vi "Playing with Octave Bands.vi"() -> ()   [LabVIEW 2014]
uses:
  <vilib>/Analysis/baseanly.llb/Mean (DBL).vi
  <vilib>/measure/maspectr.llb/FFT Spectrum (Mag-Phase) for 1 Chan.vi
  <vilib>/Analysis/NI_AALBase.lvlib
  <vilib>/Analysis/NI_AALPro.lvlib
  <vilib>/measure/NI_MAPro.lvlib
panel:
  in  "bandwidth":T1(ring)=enum."1/3 octave"
  in  "Octave":dbl=0.33 format="%#_13g"
  out "Mic Spectrum 3":cluster{"Fctr":ext[], "magnitude":dbl[]}[](graph)=[{"Fctr"=[25.73721928961165, 32.352028870043036, 40.66693298256041, 51.11887865986131, 64.25711416600414, 80.77205191484325, 101.53154954452943, 127.62651571339914, 160.428237195363, 201.66043980553155, 253.48986994750726, 318.6401568298155, 400.534938794811, 503.47777502835936, 632.87829698514, 795.5364837549187, 1000.0, 1257.0133745218284, 1580.0826237267545, 1986.1849908740721, 2496.6610978032245, 3138.3363915870036, 3944.9308179734376, 4958.830799755948, 6233.3166372840005, 7835.362380695417, 9849.155306759334, 12380.519948339124, 15562.479158596574, 19562.244443073105], "magnitude"=[-59.22433454414856, -66.2314935000544, -66.10124910819798, -73.25405372586764, -72.91725269257354, -79.52986667892496, -79.44581491850705, -83.20512373119247, -82.7593394941647, -89.63537694174055, -87.7998305536222, -89.44346376976519, -90.85831760499235, -98.17900781672215, -88.73245480537615, -88.59138292453578, -92.70765312280365, -94.03489436301587, -92.74361707931767, -94.5497480805882, -97.3842899584312, -97.20730378363506, -99.43262058496059, -102.03224809586673, -105.2012624044125, -106.33142078355012, -106.10469195235223, -106.06589607465796, -106.30619707837911, -106.64145916286945]}, {"Fctr"=array[22050 elements], "magnitude"=array[22050 elements]}]
  in  "window":u32(ring)=1 items=["Rectangle"=0, "Hanning"=1, "Hamming"=2, "Blackman-Harris"=3, "Exact Blackman"=4, "Blackman"=5, "Flat Top"=6, "4 Term B-Harris "=7, "7 Term B-Harris"=8, "Low Sidelobe"=9, "Blackman Nuttall"=11, "Triangle"=30, "Bartlett-Hanning"=31, "Bohman"=32, "Parzen"=33, "Welch"=34, "Kaiser"=60, "Dolph-Chebyshev"=61, "Gaussian"=62]
  out "Fmax":ext[](array[numeric])=[28.85569721029358, 36.271997324491245, 45.594385757505464, 57.312752700291945, 72.04289667492901, 90.55888465967992, 113.83372919899729, 143.09052007483558, 179.8666975013525, 226.09484439027202, 284.2042433090035, 357.24853493527326, 449.0661864419671, 564.4822024030656, 709.5616781001912, 891.9285194200927, 1121.1660780285088, 1409.3207551420194, 1771.5350382047216, 2226.843236457373, 2799.1717311903926, 3518.5963036897433, 4422.922613281076, 5559.67287936935, 6988.583167333556, 8784.7425102964, 11042.538827173037, 13880.618994433093, 17448.12372264413, 21932.524879675264]
  out "Fmin":ext[](array[numeric])=[22.955759894973568, 28.855697210293577, 36.27199732449124, 45.59438575750547, 57.31275270029194, 72.042896674929, 90.55888465967992, 113.83372919899729, 143.09052007483558, 179.8666975013525, 226.094844390272, 284.20424330900346, 357.2485349352732, 449.0661864419671, 564.4822024030656, 709.5616781001912, 891.9285194200927, 1121.1660780285088, 1409.3207551420196, 1771.5350382047213, 2226.843236457373, 2799.171731190392, 3518.5963036897433, 4422.922613281076, 5559.672879369349, 6988.583167333556, 8784.7425102964, 11042.538827173037, 13880.61899443309, 17448.12372264413]
  out "Fctr":ext[](array[numeric])=[25.73721928961165, 32.352028870043036, 40.66693298256041, 51.11887865986131, 64.25711416600414, 80.77205191484325, 101.53154954452943, 127.62651571339914, 160.428237195363, 201.66043980553155, 253.48986994750726, 318.6401568298155, 400.534938794811, 503.47777502835936, 632.87829698514, 795.5364837549187, 1000.0, 1257.0133745218284, 1580.0826237267545, 1986.1849908740721, 2496.6610978032245, 3138.3363915870036, 3944.9308179734376, 4958.830799755948, 6233.3166372840005, 7835.362380695417, 9849.155306759334, 12380.519948339124, 15562.479158596574, 19562.244443073105]
  in  "Upper bound":i32=20000
  in  "Lower bound":i32=20
  out "x-y":dbl=9.965784284662085
  in  "Mic Spectrum":cluster{dbl, "df":dbl, dbl[]}(graph)={0.0, "df"=1.160997732426306, array[22050 elements]}
  in  "Microphone":cluster{i32, dbl, "Data set":dbl[]}(graph)={0, 2.2675736961451248e-05, "Data set"=array[44100 elements]}
  out "error out":errorcluster
  out "octave spectrum":T2={"nominal frequencies [Hz]"=[31.5, 40.0, 50.0, 63.0, 80.0, 100.0, 125.0, 160.0, 200.0, 250.0, 315.0, 400.0, 500.0, 630.0, 800.0, 1000.0, 1250.0, 1600.0, 2000.0, 2500.0, 3150.0, 4000.0, 5000.0, 6300.0, 8000.0, 10000.0, 12500.0, 16000.0], "band power"=[-54.79091475162163, -56.58830884025793, -59.17435437723143, -58.40588122481441, -63.531004646371976, -60.32446622954747, -66.3113382355222, -65.30912585682371, -74.6827774026104, -75.5415069560743, -76.63935007180211, -77.96259672396377, -81.53215450297881, -81.36390617725992, -77.17999183733423, -78.53632587735004, -79.0266361915013, -78.93795598852955, -78.0332389362228, -77.69788600000176, -76.14179283630838, -75.47568591719252, -74.71938772039715, -73.7535091028336, -72.86644062002236, -71.9894883662107, -70.94320057402024, -69.70538283002553]} {"band power" format="%.2f"; "nominal frequencies [Hz]" format="%.2f"}
  out "XY Graph":cluster{"Fctr":ext[], "band power":dbl[]}[](graph)=[{"Fctr"=[31.5, 40.0, 50.0, 63.0, 80.0, 100.0, 125.0, 160.0, 200.0, 250.0, 315.0, 400.0, 500.0, 630.0, 800.0, 1000.0, 1250.0, 1600.0, 2000.0, 2500.0, 3150.0, 4000.0, 5000.0, 6300.0, 8000.0, 10000.0, 12500.0, 16000.0], "band power"=[-54.79091475162163, -56.58830884025793, -59.17435437723143, -58.40588122481441, -63.531004646371976, -60.32446622954747, -66.3113382355222, -65.30912585682371, -74.6827774026104, -75.5415069560743, -76.63935007180211, -77.96259672396377, -81.53215450297881, -81.36390617725992, -77.17999183733423, -78.53632587735004, -79.0266361915013, -78.93795598852955, -78.0332389362228, -77.69788600000176, -76.14179283630838, -75.47568591719252, -74.71938772039715, -73.7535091028336, -72.86644062002236, -71.9894883662107, -70.94320057402024, -69.70538283002553]}, {"Fctr"=[25.73721928961165, 32.352028870043036, 40.66693298256041, 51.11887865986131, 64.25711416600414, 80.77205191484325, 101.53154954452943, 127.62651571339914, 160.428237195363, 201.66043980553155, 253.48986994750726, 318.6401568298155, 400.534938794811, 503.47777502835936, 632.87829698514, 795.5364837549187, 1000.0, 1257.0133745218284, 1580.0826237267545, 1986.1849908740721, 2496.6610978032245, 3138.3363915870036, 3944.9308179734376, 4958.830799755948, 6233.3166372840005, 7835.362380695417, 9849.155306759334, 12380.519948339124, 15562.479158596574, 19562.244443073105], "band power"=[-59.22433454414856, -66.2314935000544, -66.10124910819798, -73.25405372586764, -72.91725269257354, -79.52986667892496, -79.44581491850705, -83.20512373119247, -82.7593394941647, -89.63537694174055, -87.7998305536222, -89.44346376976519, -90.85831760499235, -98.17900781672215, -88.73245480537615, -88.59138292453578, -92.70765312280365, -94.03489436301587, -92.74361707931767, -94.5497480805882, -97.3842899584312, -97.20730378363506, -99.43262058496059, -102.03224809586673, -105.2012624044125, -106.33142078355012, -106.10469195235223, -106.06589607465796, -106.30619707837911, -106.64145916286945]}]
  in  "Current FRF":cluster{dbl, "df":dbl, dbl[]}(graph)={0.0, "df"=1.160997732426306, array[22050 elements]}
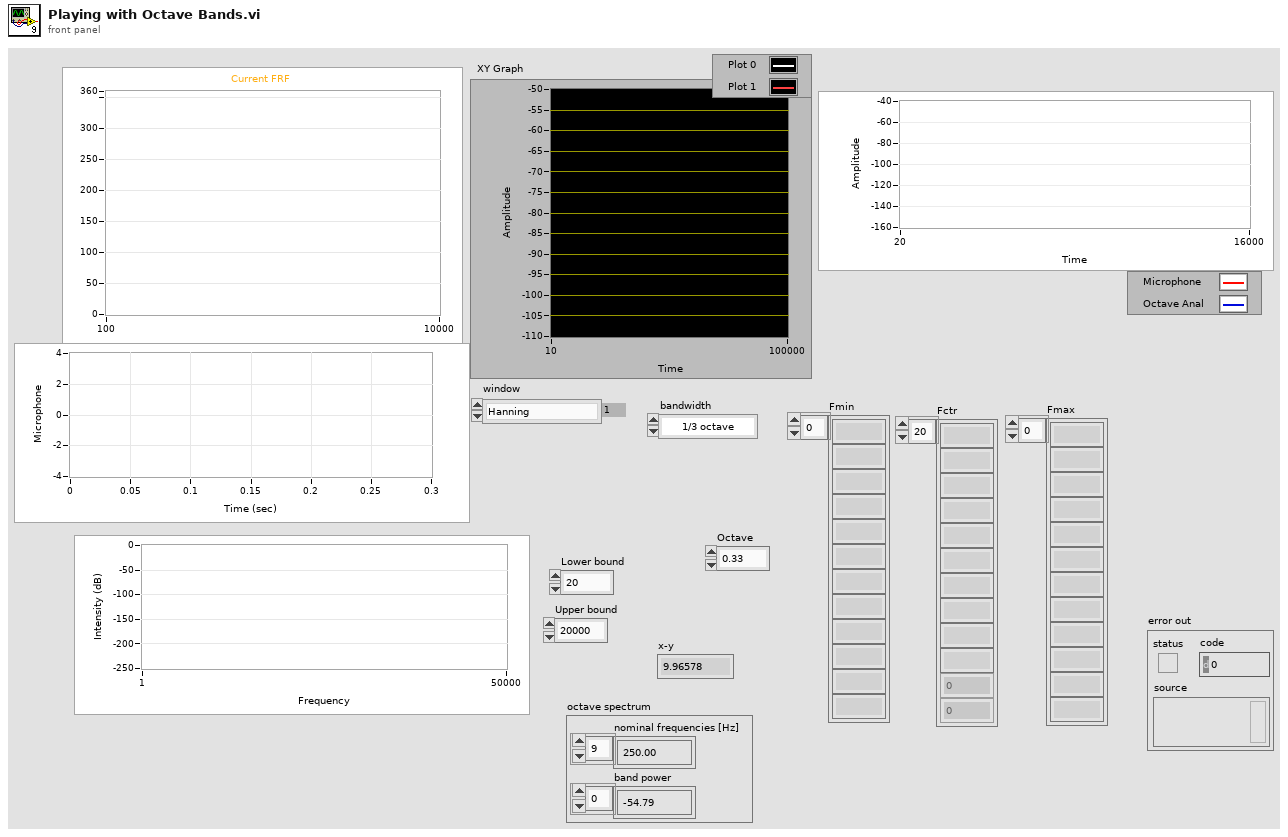
[diagram p1: front panel]
types:
  T1 = enum16{"1 octave", "1/3 octave", "1/6 octave", "1/12 octave", "1/24 octave"}
  T2 = cluster{"nominal frequencies [Hz]":dbl[], "band power":dbl[]}
  T3 = cluster{"dB On (F)":bool, "unwrap phase (F)":bool, "convert to degree (F)":bool}
  T4 = cluster{"averaging mode":enum16{"No averaging", "Vector averaging", "RMS averaging", "Peak hold"}, "weighting mode":enum16{"Linear", "Exponential"}, "number of averages":u32}
  T5 = cluster{"low band":enum16{"16 Hz", "31.5 Hz", "63 Hz", "125 Hz", "250 Hz", "500 Hz", "1000 Hz", "2000 Hz", "4000 Hz", "8000 Hz", "16000 Hz"}, "high band":enum16{"16 Hz", "31.5 Hz", "63 Hz", "125 Hz", "250 Hz", "500 Hz", "1000 Hz", "2000 Hz", "4000 Hz", "8000 Hz", "16000 Hz"}}
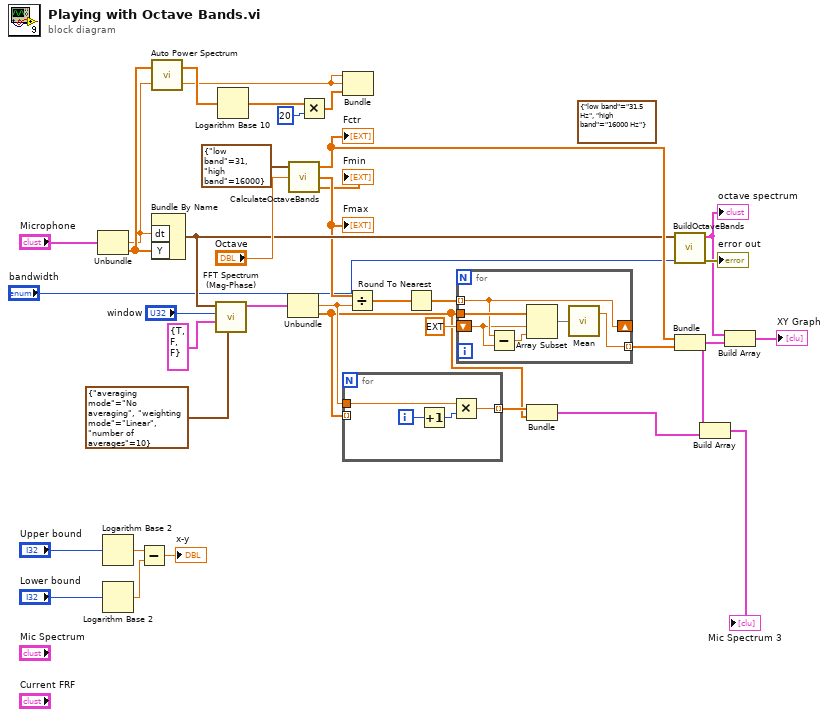
[diagram p0: block diagram]
diagram:
  (unwired) T5 {"low band"=enum."31.5 Hz", "high band"=enum."16000 Hz"} ("frequency range")
  n1 = Unbundle("Microphone") -> (w20:dbl, "Data set"=w21:dbl[])  [unwired: 1 out]
  n2 = Logarithm Base 2(1:"Upper bound") -> (0:w34:dbl)
  n3 = Logarithm Base 2(1:"Lower bound") -> (0:w35:dbl)
  n4 = Subtract(x=w34, y=w35) -> (x-y=→"x-y":dbl)
  n5 = call <vilib>:"Auto Power Spectrum.vi"("dt"=w20, "Signal (V)"=w21) -> ("df"=w18:dbl, "Power Spectrum (V^2 rms)"=w19:dbl[])
  n6 = Bundle By Name("dt"=w20, "Y"=w21) -> (w14:waveform(dbl))  [unwired: 1 in]
  n7 = call-poly <vilib>:"FFT Spectrum (Mag-Phase).vi"("averaging parameters"=T4 {"averaging mode"=enum."No averaging", "weighting mode"=enum."Linear", "number of averages"=10}, "view"=T3 {"dB On (F)"=TRUE, "unwrap phase (F)"=FALSE, "convert to degree (F)"=FALSE}, "window"="window", "time signal"=w14) -> ("magnitude"=w10:cluster{"f0":dbl, "df":dbl, "magnitude":dbl[]})  [unwired: 3 in, 4 out]
  n8 = Logarithm Base 10(1:w19) -> (0:w16:dbl[])
  n9 = Unbundle(w10) -> ("df"=w9:dbl, "magnitude"=w7:dbl[])  [unwired: 1 out]
  n10 = call <userlib>:"CalculateOctaveBands.vi"("Octave"="Octave", "frequency range"=cluster{"low band":u16, "high band":u16} {"low band"=31, "high band"=16000}) -> ("Fmin"=→"Fmin":ext[], "Fmax"=w5:ext[], "Fctr"=w25:ext[])  [unwired: 1 in]
  "Fctr" <- w25
  "Fmax" <- w5
  n11 = Multiply(x=w16, y=20) -> (x*y=w15:dbl[])
  n12 = Bundle("df"=w18, "df"=w18, w15) -> ()  [unwired: 1 in, 1 out]
  n13 = for {
    tunnel: w7 -> [_] mode=indexing
    tunnel: w9 -> [w40]
    tunnel: [w38] -> w8 mode=indexing
    i -> [w41]
    n14 = Increment(x=w41) -> (x+1=w39:i32)
    n15 = Multiply(x=w40, y=w39) -> (x*y=w38:dbl)
  }
  n16 = Divide(x=w5, y=w9) -> (x/y=w28:ext[])
  n17 = Round To Nearest(number=w28) -> (nearest integer value=w27:ext[])
  n18 = for {
    tunnel: w7 -> [w47]
    shift-right: [w46] -> _
    shift-left: ext 0.0 -> [w44]
    tunnel: w27 -> [w46] mode=indexing
    tunnel: [w42] -> w24 mode=indexing
    n19 = Subtract(x=w46, y=w44) -> (x-y=w45:ext)
    n20 = Array Subset(array=w47, index=w44, length=w45) -> (w43:dbl[])
    n21 = call-poly <vilib>:"Mean.vi"("X"=w43) -> ("mean"=w42:dbl)  [unwired: 1 out]
  }
  n22 = Bundle(w8, "magnitude"=w7) -> (w2:cluster{dbl[], "magnitude":dbl[]})  [unwired: 1 in]
  n23 = call <userlib>:"BuildOctaveBands.vi"("bandwidth"="bandwidth", "Waveform"=w14) -> ("error out"=→"error out":errorcluster, "octave spectrum"=w23:T2)  [unwired: 8 in]
  "octave spectrum" <- w23
  n24 = Bundle("Fctr"=w25, w24) -> (w1:cluster{"Fctr":ext[], dbl[]})  [unwired: 1 in]
  n25 = Build Array(w1, w2) -> (→"Mic Spectrum 3":cluster{"Fctr":ext[], "magnitude":dbl[]}[])
  n26 = Build Array(w23, w1) -> (→"XY Graph":cluster{"Fctr":ext[], "band power":dbl[]}[])
